vi "Write FIFO.vi"(8 "error in (no error)":errorcluster, 9 "timeout in ms (0)":i32 format="%d ms", 10 "element":i32, 11 "Pool in":refnum<class "Pool.lvclass">) -> (0 "error out":errorcluster, 1 "timed out?":bool, 3 "Pool out":refnum<class "Pool.lvclass">)   [LabVIEW 2017, in "Data Sharing Framework Engine.lvlib" / "Pool.lvclass"]
uses:
  Pool.lvclass
  Pool.lvclass/Pool.ctl
  Source/Data Sharing Framework Core/Engine/Debug/Debug Flags FIFO/Debug Flags FIFO.lvclass/Debug Flags FIFO.ctl
  Source/Data Sharing Framework Core/Engine/Debug/Debug Flags FIFO/Debug Flags FIFO.lvclass
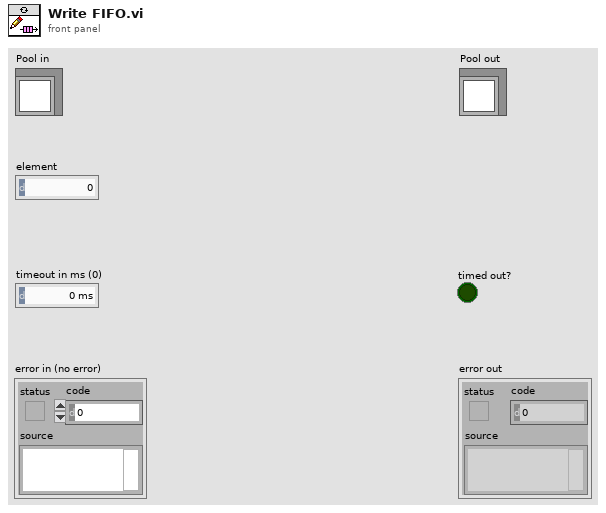
[diagram p1: front panel]
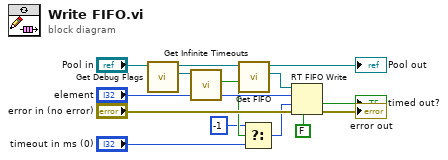
[diagram p0: block diagram]
diagram:
  n1 = call "Get Debug Flags.vi"("Pool in"="Pool in") -> ("FIFO Debug Flags"=w6:refnum<class "Debug Flags FIFO.lvclass">, "Pool out"=w1:refnum<class "Pool.lvclass">)  [unwired: 9 in]
  n2 = call "Get Infinite Timeouts.vi"("FIFO Debug Flags in"=w6) -> ("infinite timeouts"=w5:bool)  [unwired: 9 in, 1 out]
  n3 = call "Get FIFO.vi"("Pool in"=w1) -> ("FIFO"=w13:refnum<k33>, "Pool out"=→"Pool out":refnum<class "Pool.lvclass">)  [unwired: 9 in]
  n4 = Select(t=-1, s=w5, f="timeout in ms (0)") -> (s? t:f=w2:i32)
  n5 = RT FIFO Write(0:w13, 1:"element", 2:w2, 3:"error in (no error)", 5:FALSE ("overwrite on timeout (T)")) -> (10:→"timed out?":bool, 11:→"error out":errorcluster)  [unwired: 2 out]
